vi "Target Load Prosthesis Polynomials.vi"() -> (0 "Spring Polynomial":dbl[](array[numeric]), 3 "Lever Arm Polynomial":dbl[](array[numeric]))   [LabVIEW 2018, in "COBRA Prosthesis Model Library.lvlib"]
uses:
  COBRA Prosthesis Model Library.lvlib
  <vilib>/Analysis/polynomials.llb/1D Polynomial Evaluation (DBL).vi
  <vilib>/Analysis/NI_AALPro.lvlib
panel:
  out "Stiffness":cluster{"X":dbl, "Y":dbl}[](graph)
  out "Lever Arm":cluster{"X":dbl, "Y":dbl}[](graph)
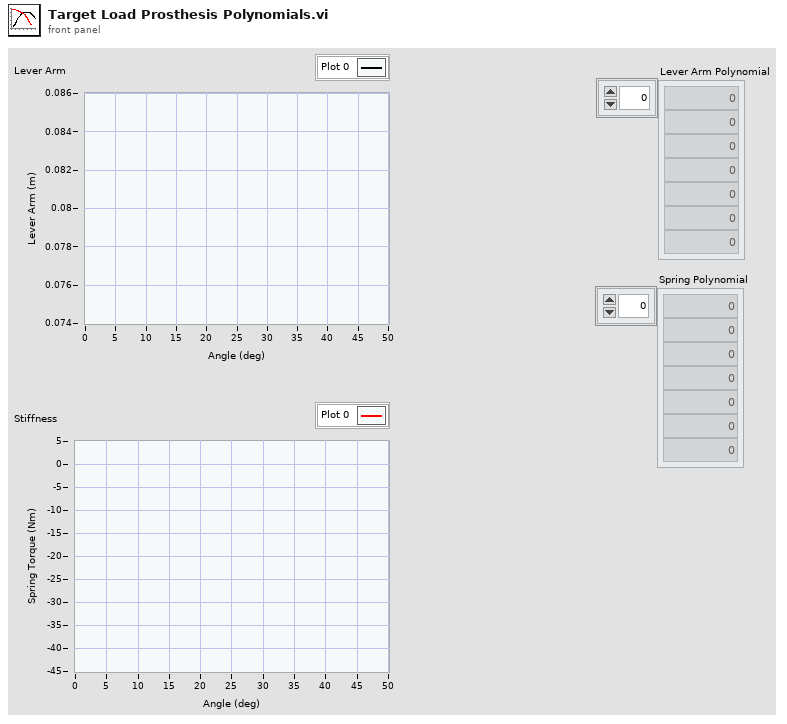
[diagram p1: front panel]
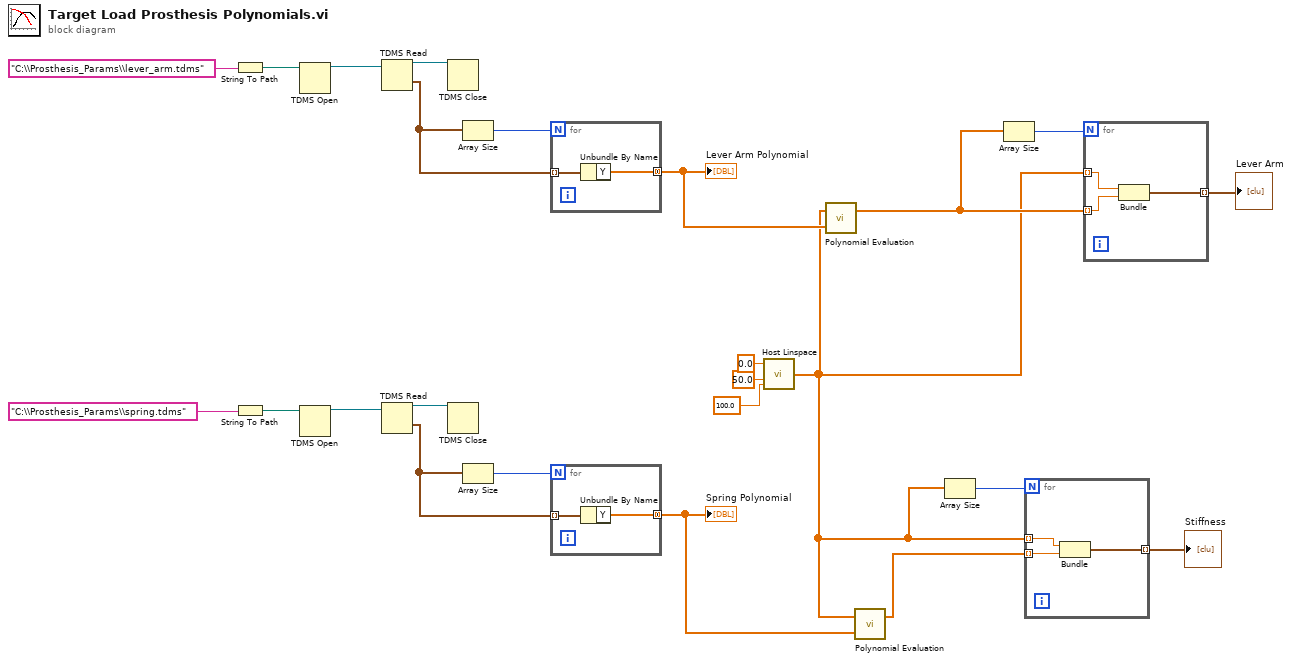
[diagram p0: block diagram]
diagram:
  n1 = String To Path(string="C:\\Prosthesis_Params\\lever_arm.tdms") -> (path=w23:path)
  n2 = String To Path(string="C:\\Prosthesis_Params\\spring.tdms") -> (path=w14:path)
  n3 = TDMS Open(11:w23) -> (3:w22:refnum<k34>)  [unwired: 6 in, 1 out]
  n4 = TDMS Open(11:w14) -> (3:w15:refnum<k34>)  [unwired: 6 in, 1 out]
  n5 = TDMS Read(0:w22) -> (4:w21:refnum<k34>, 10:w19:waveform(dbl)[])  [unwired: 7 in, 4 out]
  n6 = TDMS Read(0:w15) -> (4:w16:refnum<k34>, 10:w18:waveform(dbl)[])  [unwired: 7 in, 4 out]
  n7 = TDMS Close(11:w21) -> ()  [unwired: 1 in, 2 out]
  n8 = TDMS Close(11:w16) -> ()  [unwired: 1 in, 2 out]
  n9 = Array Size(array=w19) -> (size(s)=w20:i32)
  n10 = Array Size(array=w18) -> (size(s)=w17:i32)
  n11 = for {
    N: w20 -> [_]
    tunnel: w19 -> [w26] mode=indexing
    tunnel: [w25] -> w8 mode=concatenating
    n12 = Unbundle By Name(w26) -> ("Y"=w25:dbl[])
  }
  "Lever Arm Polynomial" <- w8
  n13 = for {
    N: w17 -> [_]
    tunnel: w18 -> [w28] mode=indexing
    tunnel: [w27] -> w5 mode=concatenating
    n14 = Unbundle By Name(w28) -> ("Y"=w27:dbl[])
  }
  "Spring Polynomial" <- w5
  n15 = call "Host Linspace.vi"("NumElements"=100.0, "End"=50.0, "Start"=0.0) -> ("Array"=w1:dbl[])
  n16 = call-poly <vilib>:"Polynomial Evaluation.vi"("P(x)"=w8, "A"=w1) -> ("P(A)"=w2:dbl[])  [unwired: 1 out]
  n17 = call-poly <vilib>:"Polynomial Evaluation.vi"("P(x)"=w5, "A"=w1) -> ("P(A)"=w4:dbl[])  [unwired: 1 out]
  n18 = Array Size(array=w1) -> (size(s)=w6:i32)
  n19 = Array Size(array=w2) -> (size(s)=w12:i32)
  n20 = for {
    N: w6 -> [_]
    tunnel: [w31] -> w3 mode=indexing
    tunnel: w4 -> [w30] mode=indexing
    tunnel: w1 -> [w29] mode=indexing
    n21 = Bundle("Numeric"=w29, "p(x)"=w30) -> (w31:cluster{"Numeric":dbl, "p(x)":dbl})  [unwired: 1 in]
  }
  "Stiffness" <- w3
  n22 = for {
    N: w12 -> [_]
    tunnel: w2 -> [w33] mode=indexing
    tunnel: w1 -> [w34] mode=indexing
    tunnel: [w32] -> w7 mode=indexing
    n23 = Bundle("Numeric"=w34, "p(x)"=w33) -> (w32:cluster{"Numeric":dbl, "p(x)":dbl})  [unwired: 1 in]
  }
  "Lever Arm" <- w7
